vi "_PC_Spectrafilter get_rectangle_position.vi"(8 "error in (no error)":errorcluster, 10 "Coords":T1, 11 "xy graph ref":refnum<vi>) -> (0 "error out":errorcluster, 1 "max value":dbl, 2 "min value":dbl)   [LabVIEW 2016]
uses:
  <vilib>/Utility/miscctls.llb/LVPoint32TypeDef.ctl
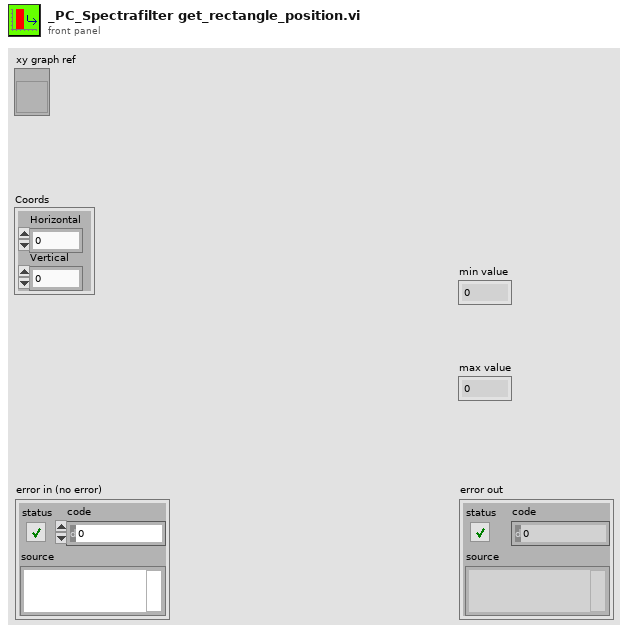
[diagram p1: front panel]
types:
  T1 = typedef "LVPoint32TypeDef.ctl" = cluster{"Horizontal":i32, "Vertical":i32}
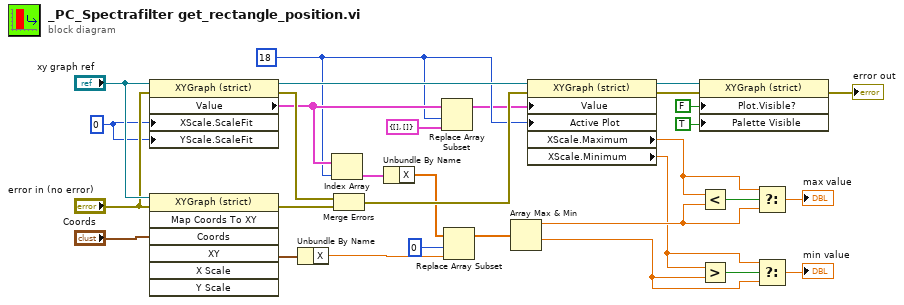
[diagram p0: block diagram]
diagram:
  w9 = u8 0 ("X Scale.Scale Fit")
  w17 = 18 ("index")
  n1 = property class="XYGraph (strict)"(reference="xy graph ref", error in="error in (no error)", "XScale.ScaleFit"=w9, "YScale.ScaleFit"=w9) -> (reference out=w29:refnum<vi>, error out=w27:errorcluster, "Value"=w19:cluster{"X":dbl[], "Y":sgl[]}[])
  n2 = invoke class="XYGraph (strict)" method="Map Coords To XY"(reference="xy graph ref", error in="error in (no error)", "Coords"="Coords") -> (error out=w28:errorcluster, "XY"=w25:cluster{"X":dbl, "Y":dbl})  [unwired: 4 in, 5 out]
  n3 = Unbundle By Name(w25) -> ("X"=w21:dbl)
  n4 = Index Array(array=w19, index=w17) -> (element=w20:cluster{"X":dbl[], "Y":sgl[]})
  n5 = Merge Errors(w27, w28) -> (w26:errorcluster)
  n6 = Unbundle By Name(w20) -> ("X"=w23:dbl[])
  n7 = Replace Array Subset(array=w19, new element=cluster{"X":dbl[], "Y":sgl[]} {"X"=[], "Y"=[]} ("new element/subarray"), index=w17) -> (w16:cluster{"X":dbl[], "Y":sgl[]}[])
  n8 = Replace Array Subset(array=w23, new element=w21, index=0) -> (w18:dbl[])
  n9 = Array Max & Min(array=w18) -> (max value=w6:dbl, min value=w2:dbl)  [unwired: 2 out]
  n10 = property class="XYGraph (strict)"(reference=w29, error in=w26, "Value"=w16, "Active Plot"=w17) -> (reference out=w13:refnum<vi>, error out=w12:errorcluster, "XScale.Maximum"=w7:dbl, "XScale.Minimum"=w3:dbl)
  n11 = property class="XYGraph (strict)"(reference=w13, error in=w12, "Plot.Visible?"=FALSE ("Visible"), "Palette Visible"=TRUE ("Palette:Visible")) -> (error out=→"error out":errorcluster)  [unwired: 1 out]
  n12 = Less?(x=w7, y=w6) -> (x < y?=w8:bool)
  n13 = Greater?(x=w3, y=w2) -> (0:w4:bool)
  n14 = Select(t=w7, s=w8, f=w6) -> (s? t:f=→"max value":dbl)
  n15 = Select(t=w3, s=w4, f=w2) -> (s? t:f=→"min value":dbl)
